vi "Conf_DI.vi"(8 "error in (no error)":errorcluster, 10 "PIN Number":i8, 11 "DI_DO in":refnum<class "DI_DO.lvclass">) -> (0 "error out":errorcluster, 3 "DI_DO out":refnum<class "DI_DO.lvclass">)   [LabVIEW 2023, in "Driver_DI_DO.lvlib" / "DI_DO.lvclass"]
uses:
  DI_DO.lvclass
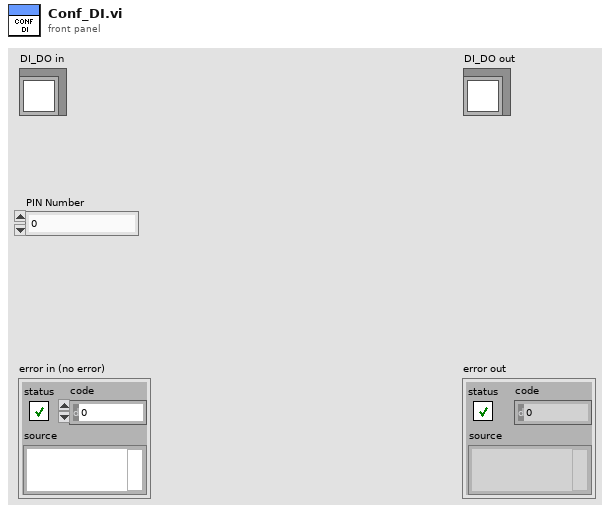
[diagram p1: front panel]
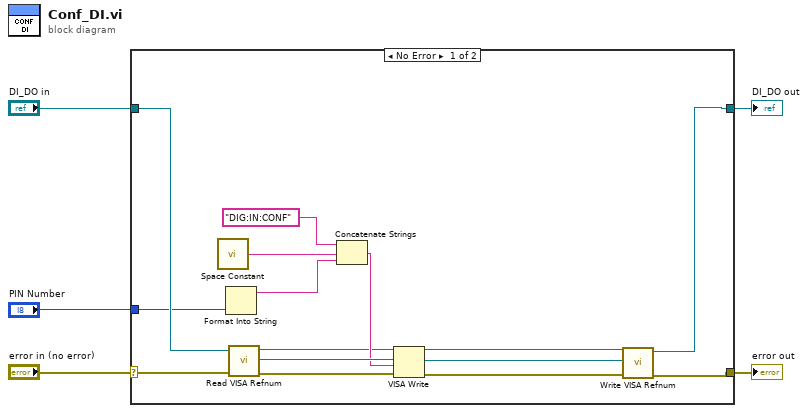
[diagram p0: block diagram]
diagram:
  n1 = case shown="No Error" "error in (no error)" {
    selector: "error in (no error)" -> [w13 w21]
    tunnel: [w11 w21] -> w4
    tunnel: [w10 w20] -> w2
    tunnel: "DI_DO in" -> [w9 w20]
    tunnel: "PIN Number" -> [w6 _]
    frame No Error {
      n2 = call <vilib>:"Space Constant.vi"() -> ("String"=w18:string)
      n3 = Format Into String(w6) -> (resulting string=w17:string)  [unwired: 3 in, 1 out]
      n4 = call-dynamic "Read VISA Refnum.vi"("error in (no error)"=w13, "Driver in"=w9) -> ("error out"=w14:errorcluster, "VISA Refnum"=w16:refnum<visa-resource-name>, "Driver out"=w8:refnum<class "DI_DO.lvclass">)  [unwired: 7 in]
      n5 = Concatenate Strings("DIG:IN:CONF", w18, w17) -> (w15:string)
      n6 = VISA Write(VISA resource name=w16, write buffer=w15, error in (no error)=w14) -> (VISA resource name out=w7:refnum<visa-resource-name>, error out=w12:errorcluster)  [unwired: 1 out]
      n7 = call-dynamic "Write VISA Refnum.vi"("error in (no error)"=w12, "VISA Refnum"=w7, "Driver in"=w8) -> ("error out"=w11:errorcluster, "Driver out"=w10:refnum<class "DI_DO.lvclass">)  [unwired: 7 in]
    }
    frame Error {
    }
  }
  "error out" <- w4
  "DI_DO out" <- w2
